vi "Run Transient Capture Demonstration (Multiple Units).vi"() -> ()   [LabVIEW 2017]
doc: "Run a demonstration using a device driver, with the data shared across a local network.\n\nUses a configurable GUI, with multiple tabs and active plots."
uses:
  GUI/Plots/Plot Data - Main GUI.vi
  GUI/Plots/DTacq Plot Display Library.lvlib
  DTACQ - Network Enabled Device Driver.lvlib
panel:
  in  "INI Files":path[](array[path])
  in  "Maximum Waveforms per Second":dbl=1000.0
  in  "Soft Trigger":bool
  in  "Start Button":bool
  in  "Waveform Length (Samples)":i32=1000
  # "Transient Capture"
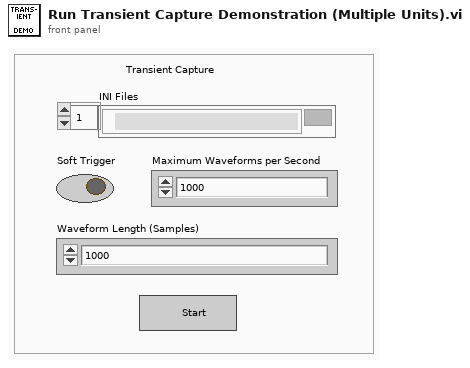
[diagram p1: front panel]
types:
  T1 = enum32{"Invalid", "Standard", "Closed", "Hidden", "Minimized", "Maximized"}
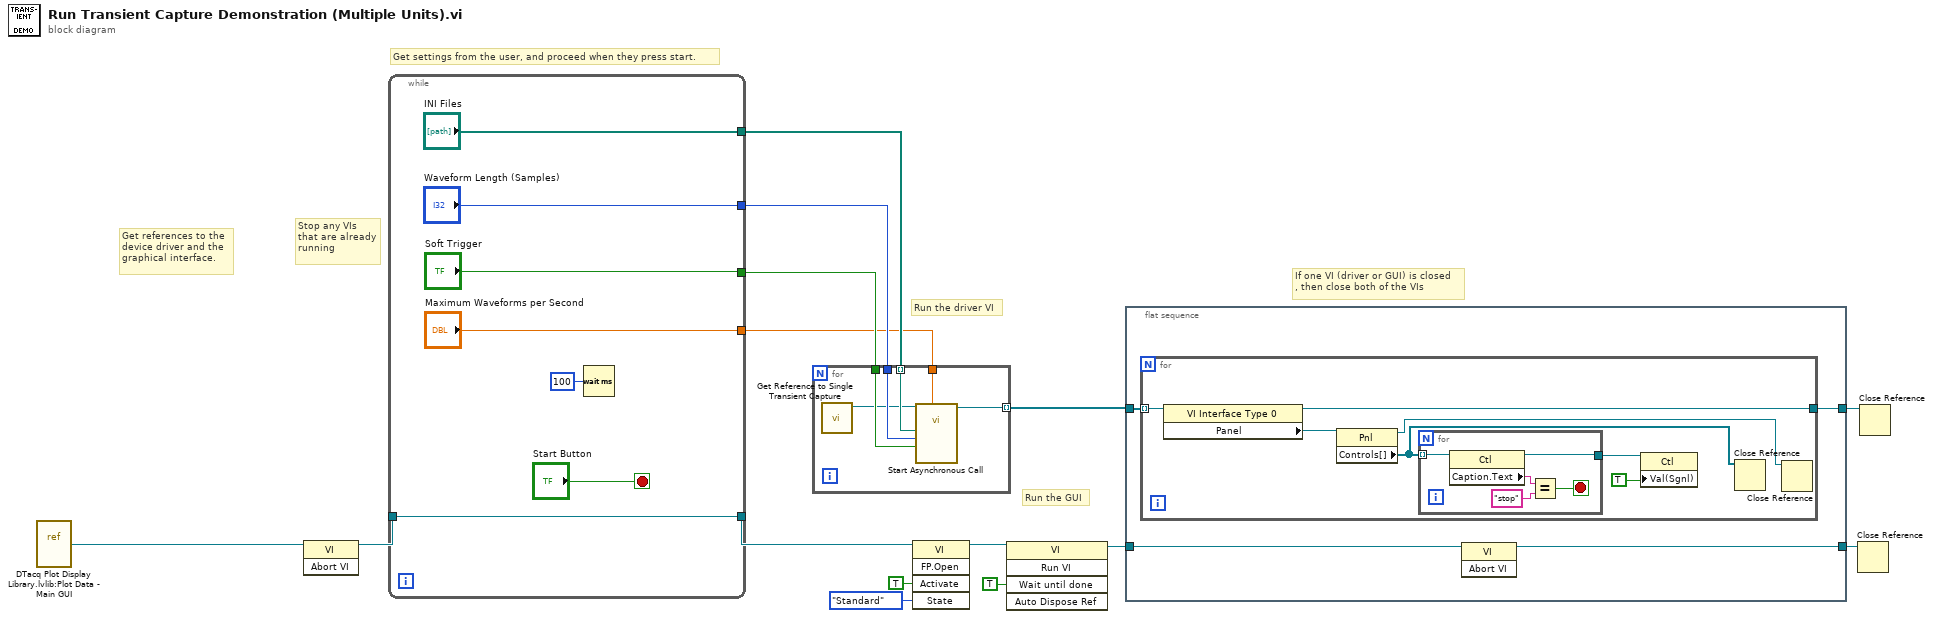
[diagram p0: block diagram]
diagram:
  # "If one VI (driver or GUI) is closed\n, then close both of the VIs"
  # "Run the GUI"
  # "Run the driver VI"
  # "Get settings from the user, and proceed when they press start."
  # "Stop any VIs\nthat are already\nrunning"
  # "Get references to the\ndevice driver and the\ngraphical interface."
  n1 = vi-ref "DTacq Plot Display Library.lvlib:Plot Data - Main GUI.vi"() -> (w13:refnum<vi>)
  n2 = invoke class="VI" method="Abort VI"(reference=w13) -> (reference out=w5:refnum<vi>)  [unwired: 2 in, 2 out]
  n3 = while {
    tunnel: ["INI Files"] -> w7
    tunnel: ["Waveform Length (Samples)"] -> w6
    tunnel: w5 -> [w21]
    tunnel: [w21] -> w4
    tunnel: ["Soft Trigger"] -> w3
    tunnel: ["Maximum Waveforms per Second"] -> w2
    stop <- "Start Button" stop-if-true
    n4 = Wait (ms)(milliseconds to wait=u32 100) -> ()  [unwired: 1 out]
  }
  n5 = for {
    tunnel: w7 -> [w28] mode=indexing
    tunnel: w6 -> [w27]
    tunnel: w3 -> [w26]
    tunnel: w2 -> [w25]
    tunnel: [w23] -> w1 mode=indexing
    n6 = call "Get Reference to Single Transient Capture.vi"() -> ("VI out"=w24:refnum<vi>)  [unwired: 11 in]
    n7 = call-by-ref "Start Asynchronous Call"(reference=w24, "Maximum Waveforms/Second"=w25, "Soft Trigger"=w26, "Maximum Waveform Length"=w27, "configuration file path"=w28) -> (reference out=w23:refnum<vi>)  [unwired: 8 in, 2 out]
  }
  n8 = invoke class="VI" method="FP.Open"(reference=w4, "Activate"=TRUE ("Activate?"), "State"=T1."Standard") -> (reference out=w12:refnum<vi>)  [unwired: 2 in, 4 out]
  n9 = invoke class="VI" method="Run VI"(reference=w12, "Wait until done"=TRUE ("Wait Until Done")) -> (reference out=w10:refnum<vi>)  [unwired: 3 in, 4 out]
  n10 = flat-sequence {
    tunnel: w1 -> [w30]
    tunnel: w10 -> [w32]
    tunnel: [w31] -> w9
    tunnel: [w29] -> w8
    frame #0 {
      n11 = for {
        tunnel: w30 -> [w39] mode=indexing
        tunnel: [w33] -> w29
        n12 = property class="VI Interface Type 0"(reference=w39) -> (reference out=w33:refnum<vi>, "Panel"=w38:refnum<vi>)  [unwired: 1 in, 1 out]
        n13 = property class="Pnl"(reference=w38) -> (reference out=w34:refnum<vi>, "Controls[]"=w35:refnum<vi>[])  [unwired: 1 in, 1 out]
        n14 = for {
          tunnel: w35 -> [w44] mode=indexing
          tunnel: [w40] -> w37
          stop <- w41 stop-if-true
          n15 = property class="Ctl"(reference=w44) -> (reference out=w40:refnum<vi>, "Caption.Text"=w43:string)  [unwired: 1 in, 1 out]
          n16 = Equal?(x=w43, y="stop") -> (x = y?=w41:bool)
        }
        n17 = property class="Ctl"(reference=w37, "Val(Sgnl)"=TRUE) -> ()  [unwired: 1 in, 2 out]
        n18 = Close Reference(reference=w35) -> ()  [unwired: 1 in, 1 out]
        n19 = Close Reference(reference=w34) -> ()  [unwired: 1 in, 1 out]
      }
      n20 = invoke class="VI" method="Abort VI"(reference=w32) -> (reference out=w31:refnum<vi>)  [unwired: 2 in, 2 out]
    }
  }
  n21 = Close Reference(reference=w9) -> ()  [unwired: 1 in, 1 out]
  n22 = Close Reference(reference=w8) -> ()  [unwired: 1 in, 1 out]
